vi "Hardnass_ClusterToString_Array.vi"(0 "Hardness_test":T1, 5 "Hardness_test 2":T1, 7 "Hardness_test 3":T1, 9 "Hardness_test 4":T1, 11 "Hardness_test 5":T1) -> (8 "StringArray":string[](array[string]))   [LabVIEW 2019]
uses:
  Hardness_test.ctl
  TEST.lvclass
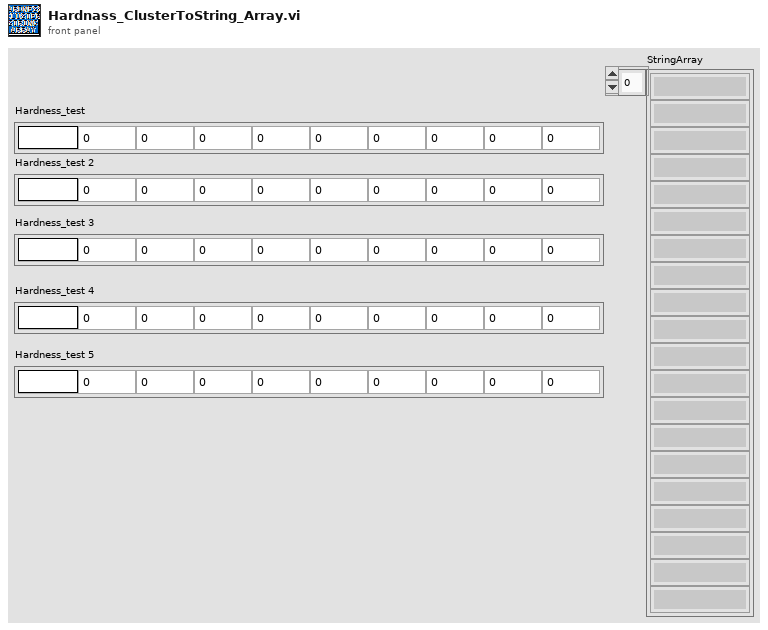
[diagram p1: front panel]
types:
  T1 = typedef "TEST.lvclass/Hardness_test.ctl" = cluster{"HN":string, "HS":sgl, "TV1":sgl, "TV2":sgl, "TV3":sgl, "TV4":sgl, "TV5":sgl, "AVG":sgl, "HV":sgl, "REP":sgl}
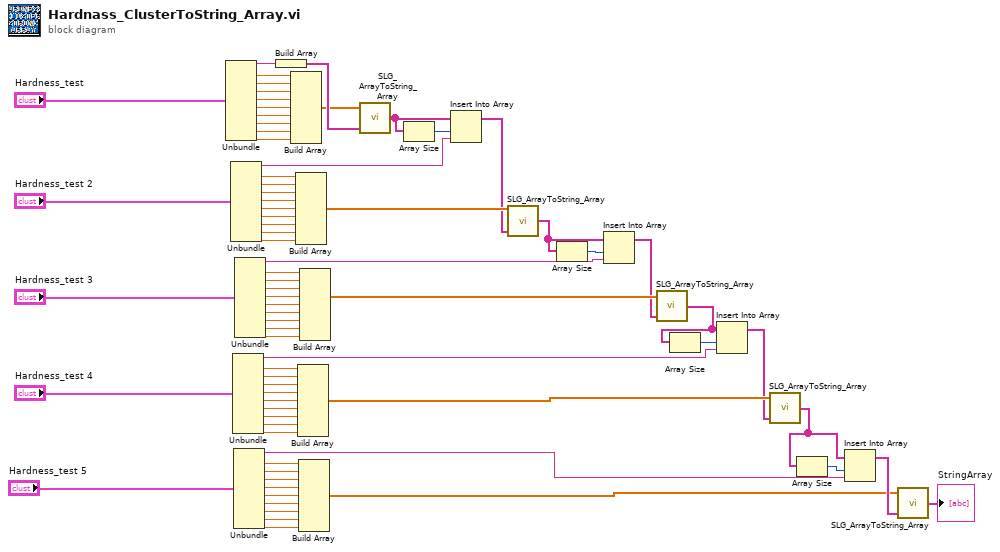
[diagram p0: block diagram]
diagram:
  n1 = Unbundle("Hardness_test") -> ("HN"=w73:string, "HS"=w71:sgl, "TV1"=w70:sgl, "TV2"=w69:sgl, "TV3"=w68:sgl, "TV4"=w67:sgl, "TV5"=w66:sgl, "AVG"=w65:sgl, "HV"=w64:sgl, "REP"=w63:sgl)
  n2 = Unbundle("Hardness_test 2") -> ("HN"=w17:string, "HS"=w52:sgl, "TV1"=w53:sgl, "TV2"=w54:sgl, "TV3"=w55:sgl, "TV4"=w56:sgl, "TV5"=w57:sgl, "AVG"=w58:sgl, "HV"=w59:sgl, "REP"=w60:sgl)
  n3 = Unbundle("Hardness_test 4") -> ("HN"=w7:string, "HS"=w33:sgl, "TV1"=w34:sgl, "TV2"=w35:sgl, "TV3"=w36:sgl, "TV4"=w37:sgl, "TV5"=w38:sgl, "AVG"=w39:sgl, "HV"=w40:sgl, "REP"=w41:sgl)
  n4 = Unbundle("Hardness_test 5") -> ("HN"=w4:string, "HS"=w32:sgl, "TV1"=w31:sgl, "TV2"=w30:sgl, "TV3"=w29:sgl, "TV4"=w28:sgl, "TV5"=w27:sgl, "AVG"=w26:sgl, "HV"=w25:sgl, "REP"=w24:sgl)
  n5 = Unbundle("Hardness_test 3") -> ("HN"=w13:string, "HS"=w51:sgl, "TV1"=w50:sgl, "TV2"=w49:sgl, "TV3"=w48:sgl, "TV4"=w47:sgl, "TV5"=w46:sgl, "AVG"=w45:sgl, "HV"=w44:sgl, "REP"=w43:sgl)
  n6 = Build Array(w73) -> (w72:string[])
  n7 = Build Array(w71, w70, w69, w68, w67, w66, w65, w64, w63) -> (w62:sgl[])
  n8 = Build Array(w52, w53, w54, w55, w56, w57, w58, w59, w60) -> (w61:sgl[])
  n9 = Build Array(w33, w34, w35, w36, w37, w38, w39, w40, w41) -> (w6:sgl[])
  n10 = Build Array(w32, w31, w30, w29, w28, w27, w26, w25, w24) -> (w3:sgl[])
  n11 = Build Array(w51, w50, w49, w48, w47, w46, w45, w44, w43) -> (w42:sgl[])
  n12 = call "SLG_ArrayToString_Array.vi"("OrArray"=w72, "SLG_Array"=w62) -> ("StringArray"=w19:string[])  [unwired: 1 in]
  n13 = Array Size(array=w19) -> (size(s)=w18:i32)
  n14 = Insert Into Array(array=w19, index=w18, new element=w17) -> (w16:string[])
  n15 = call "SLG_ArrayToString_Array.vi"("OrArray"=w16, "SLG_Array"=w61) -> ("StringArray"=w14:string[])  [unwired: 1 in]
  n16 = Array Size(array=w14) -> (size(s)=w15:i32)
  n17 = Insert Into Array(array=w14, index=w15, new element=w13) -> (w12:string[])
  n18 = call "SLG_ArrayToString_Array.vi"("OrArray"=w12, "SLG_Array"=w42) -> ("StringArray"=w8:string[])  [unwired: 1 in]
  n19 = Array Size(array=w8) -> (size(s)=w11:i32)
  n20 = Insert Into Array(array=w8, index=w11, new element=w7) -> (w1:string[])
  n21 = call "SLG_ArrayToString_Array.vi"("OrArray"=w1, "SLG_Array"=w6) -> ("StringArray"=w5:string[])  [unwired: 1 in]
  n22 = Array Size(array=w5) -> (size(s)=w10:i32)
  n23 = Insert Into Array(array=w5, index=w10, new element=w4) -> (w9:string[])
  n24 = call "SLG_ArrayToString_Array.vi"("OrArray"=w9, "SLG_Array"=w3) -> ("StringArray"=→"StringArray":string[])  [unwired: 1 in]
